vi "New VI.vi"() -> ()   [LabVIEW 2015]
panel:
  in  "Stop Button":bool
  out "Boolean":bool
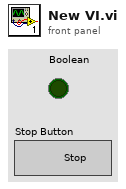
[diagram p1: front panel]
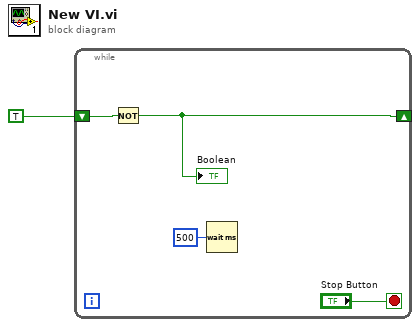
[diagram p0: block diagram]
diagram:
  n1 = while {
    shift-right: [w4] -> _
    shift-left: TRUE -> [w5]
    stop <- "Stop Button" stop-if-true
    n2 = Not(x=w5) -> (.not. x?=w4:bool)
    "Boolean" <- w4
    n3 = Wait (ms)(milliseconds to wait=u32 500) -> ()  [unwired: 1 out]
  }
